vi "show data.vi"(8 "error in (no error)":errorcluster, 11 "DataTypes in":refnum<class "DataTypes.lvclass">) -> (0 "error out":errorcluster, 3 "DataTypes out":refnum<class "DataTypes.lvclass">)   [LabVIEW 2018, in "DataTypes.lvclass"]
uses:
  DataTypes.lvclass
  DataTypes.lvclass/DataTypes.ctl
panel:
  out "Ring 2":u16(ring)=1 items=["ring-item-0", "ring-item-1", "ring-item-2"]
  out "Time Stamp":timestamp
  out "Numeric I64":i64
  out "Numeric U64":u64
  out "Numeric I32":i32
  out "Numeric U32":u32
  out "Numeric I16":i16
  out "Numeric U16":u16
  out "Numeric I8":i8
  out "Numeric U8":u8
  out "Numeric C-SGL":csg
  out "Numeric C-DBL":cdb
  out "Numeric SGL":sgl
  out "Numeric DBL":dbl
  out "Enum":T1(ring)
  out "Ring":u16
  out "String":string
  out "Boolean":bool
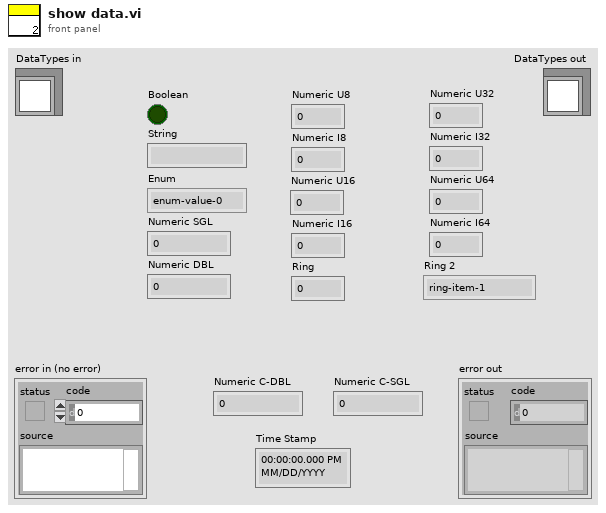
[diagram p1: front panel]
types:
  T1 = enum16{"enum-value-0", "enum-value-1", "enum-value-2"}
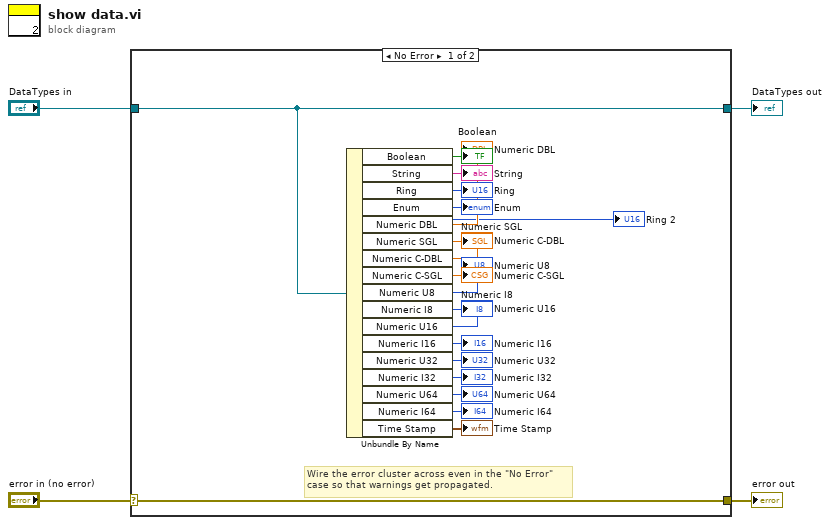
[diagram p0: block diagram]
diagram:
  n1 = case shown="No Error" "error in (no error)" {
    selector: "error in (no error)" -> [w23 w25]
    tunnel: [w23 w25] -> w3
    tunnel: [w22 w24] -> w1
    tunnel: "DataTypes in" -> [w22 w24]
    frame No Error {
      # "Wire the error cluster across even in the \"No Error\"\ncase so that warnings get propagated."
      n2 = Unbundle By Name(w22) -> ("Boolean"=→"Boolean":bool, "String"=→"String":string, "Ring"=→"Ring" →"Ring 2":u16, "Enum"=→"Enum":T1, "Numeric DBL"=→"Numeric DBL":dbl, "Numeric SGL"=→"Numeric SGL":sgl, "Numeric C-DBL"=→"Numeric C-DBL":cdb, "Numeric C-SGL"=→"Numeric C-SGL":csg, "Numeric U8"=→"Numeric U8":u8, "Numeric I8"=→"Numeric I8":i8, "Numeric U16"=→"Numeric U16":u16, "Numeric I16"=→"Numeric I16":i16, "Numeric U32"=→"Numeric U32":u32, "Numeric I32"=→"Numeric I32":i32, "Numeric U64"=→"Numeric U64":u64, "Numeric I64"=→"Numeric I64":i64, "Time Stamp"=→"Time Stamp":timestamp)
    }
    frame Error {
    }
  }
  "error out" <- w3
  "DataTypes out" <- w1
